vi "Open VISA Ref.vi"(8 "ErrorIn":errorcluster, 10 "BaudRate":u32=9600, 11 "VISAResourceName":refnum<visa-resource-name>) -> (0 "ErrorOut":errorcluster, 3 "VISA resource name out":refnum<visa-resource-name>)   [LabVIEW 2017, in "I28Drivers.lvlib"]
uses:
  I28Drivers.lvlib
  <vilib>/Instr/_visa.llb/VISA Configure Serial Port (Instr).vi
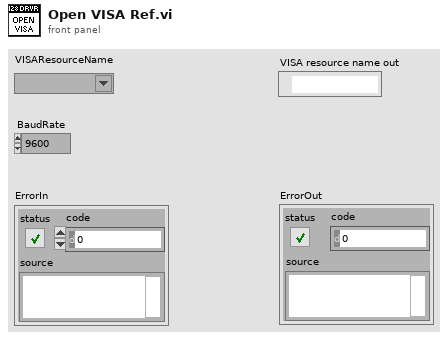
[diagram p1: front panel]
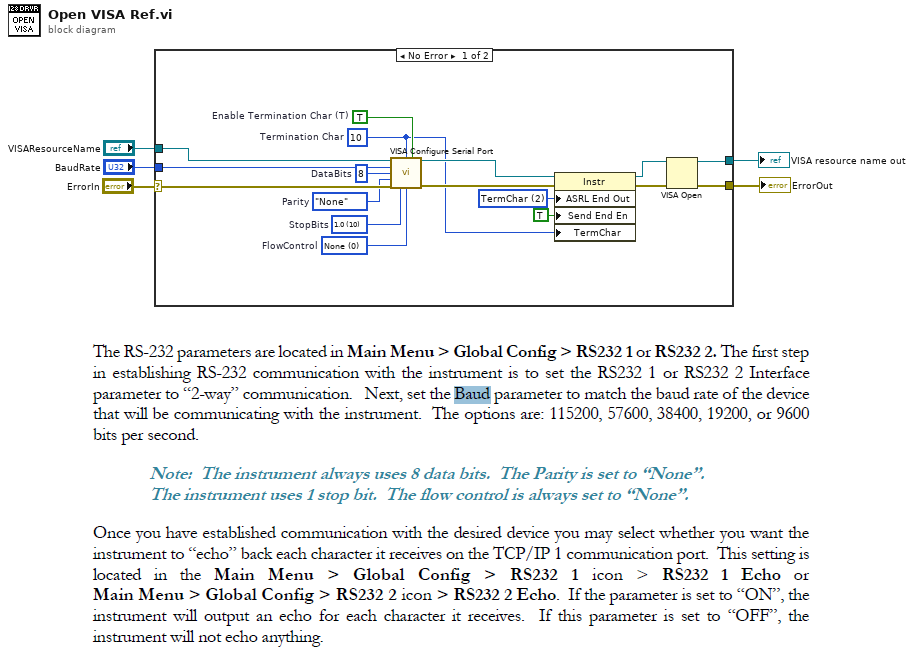
[diagram p0: block diagram]
diagram:
  n1 = case shown="No Error" "ErrorIn" {
    selector: "ErrorIn" -> [w21 w24]
    tunnel: "VISAResourceName" -> [w22 w23]
    tunnel: "BaudRate" -> [w20 _]
    tunnel: [w8 w24] -> w2
    tunnel: [w7 w23] -> w3
    frame No Error {
      w14 = u16 2 items=["None", "Last Bit", "TermChar", "Break"] ("Serial Settings:End Mode for Writes")
      w15 = u16 0 items=["None", "XON/XOFF", "RTS/CTS", "XON/XOFF & RTS/CTS", "DTR/DSR", "XON/XOFF & DTR/DSR"]  # FlowControl
      w16 = u16 10 items=["1.0"=10, "1.5"=15, "2.0"=20]  # StopBits
      w17 = TRUE  # Enable Termination Char (T)
      w6 = u8 10  # Termination Char
      w18 = enum16{"None", "Odd", "Even", "Mark", "Space"}."None"  # Parity
      w19 = u16 8  # DataBits
      n2 = call-poly "VISA Configure Serial Port"("VISA resource name"=w22, "termination char\n(0xA = '\\n' = LF)"=w6, "Enable Termination\nChar (T)"=w17, "baud rate (9600)"=w20, "data bits (8)"=w19, "parity (0:none)"=w18, "error in (no error)"=w21, "stop bits (10: 1 bit)"=w16, "flow control (0:none)"=w15) -> ("VISA resource name out"=w11:refnum<visa-resource-name>, "error out"=w12:errorcluster)  [unwired: 5 in]
      n3 = property class="Instr"(reference=w11, error in=w12, "ASRL End Out"=w14, "Send End En"=TRUE ("Message Based Settings:Send End Enable"), "TermChar"=w6) -> (reference out=w9:refnum<visa-resource-name>, error out=w10:errorcluster)
      n4 = VISA Open(error in (no error)=w10, VISA resource name=w9) -> (VISA resource name=w7:refnum<visa-resource-name>, error out=w8:errorcluster)  [unwired: 3 in]
    }
    frame Error {
    }
  }
  "VISA resource name out" <- w3
  "ErrorOut" <- w2
